vi "反控参数变更.vi"(11 "设置参数":T1(ring)=enum."CODMn") -> ()   [LabVIEW 2016, in "斯坦道CODMn新电路板.lvlib"]
panel:
  in  "错误输入（无错误）":errorcluster
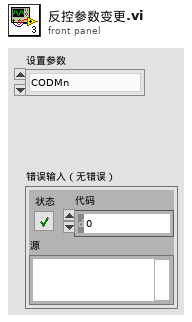
[diagram p1: front panel]
types:
  T1 = enum16{"", "CODMn", "PH", "氨氮", "总氮", "总磷", "CODCr", "电导率", "水温", "溶解氧", "浊度", "叶绿素", "藻密度", "ORP"}
  T2 = typedef "量程选择控件.ctl" = enum32{"L", "H", "AUTO"}
  T3 = typedef "操作日志字段定义.ctl" = cluster{"时间":timestamp, "参数":string, "日志信息":string, "流程参数":string}
  T4 = cluster{"水样测试量程模式":T2, "标样核查量程模式":T2, "零点核查量程模式":T2, "跨度核查量程模式":T2, "空白测试量程模式":T2, "平行样测试量程模式":T2, "加标回收量程模式":T2, "空白校准量程模式":T2, "标样校准量程模式":T2}
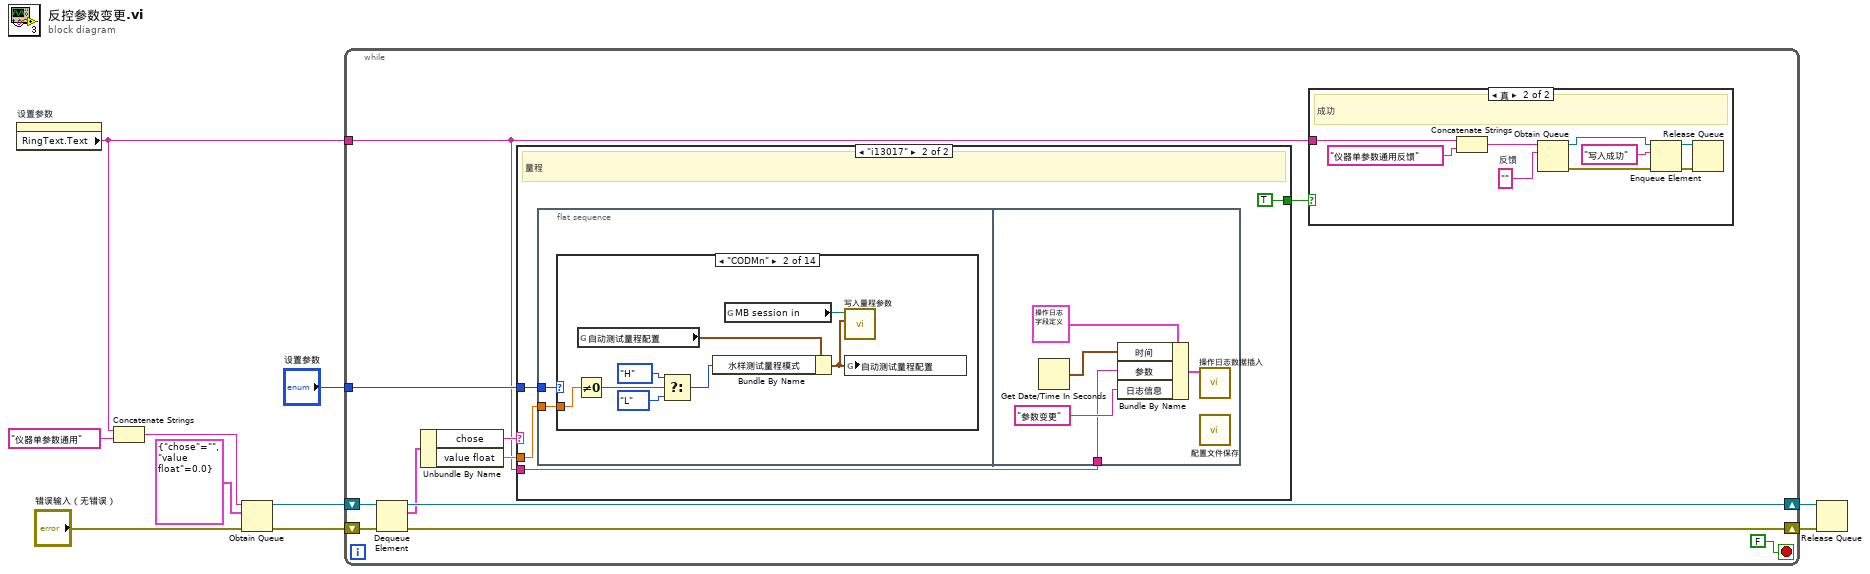
[diagram p0: block diagram]
diagram:
  n1 = property on="设置参数" class="Enum (严格)"() -> ("RingText.Text"=w2:string)  [unwired: 2 in, 2 out]
  n2 = Concatenate Strings(w2, "仪器单参数通用" ("名称（未命名）")) -> (w7:string)
  n3 = Obtain Queue(name (unnamed)=w7, element data type=cluster{"chose":string, "value float":dbl} {"chose"="", "value float"=0.0}, error in (no error)="错误输入（无错误）") -> (queue out=w6:refnum<queue>, error out=w5:errorcluster)  [unwired: 2 in, 1 out]
  n4 = while {
    shift-right: [w19] -> w4
    shift-left: w6 -> [w21]
    shift-right: [w18] -> w3
    shift-left: w5 -> [w20]
    tunnel: w2 -> [w11]
    tunnel: "设置参数" -> [w12]
    stop <- FALSE stop-if-true
    n5 = Dequeue Element(queue=w21, error in (no error)=w20) -> (queue out=w19:refnum<queue>, element=w16:cluster{"chose":string, "value float":dbl}, error out=w18:errorcluster)  [unwired: 1 in, 1 out]
    n6 = Unbundle By Name(w16) -> ("chose"=w15:string, "value float"=w13:dbl)
    n7 = case shown="\"i13017\"" w15 {
      tunnel: w13 -> [_ w32]
      tunnel: [_ TRUE] -> w14
      tunnel: w12 -> [_ w33]
      tunnel: w11 -> [_ w31]
      frame "假", Default {
      }
      frame "i13017" {
        # "量程"
        n8 = flat-sequence {
          tunnel: w33 -> [w36]
          tunnel: w32 -> [w35]
          tunnel: w31 -> [w46]
          frame #0 {
            n9 = case shown="\"CODMn\"" w36 {
              tunnel: w35 -> [_ w44 _ _ _ _ _ _ _ _ _ _ _ _]
              frame "", Default {
              }
              frame "CODMn" {
                n10 = Not Equal To 0?(x=w44) -> (x != 0?=w43:bool)
                n11 = global read "CODMn断电保存全局变量.vi" "自动测试量程配置"() -> (w40:T4)
                n12 = Select(t=量程选择控件."H" ("水样测试量程模式"), s=w43, f=量程选择控件."L" ("水样测试量程模式")) -> (s? t:f=w37:T2)
                n13 = Bundle By Name(cluster=w40, "水样测试量程模式"=w37) -> (w41:T4)
                n14 = global read "VARCODMn全局变量.vi" "MB session in"() -> (w39:refnum<class "MB_Master.lvclass">)
                n15 = call "写入量程参数.vi"("自动测试量程配置"=w41, "MB session in"=w39) -> ()  [unwired: 8 in, 2 out]
                n16 = global write "CODMn断电保存全局变量.vi" "自动测试量程配置"(w41) -> ()
              }
              frame "PH" {
              }
              frame "氨氮" {
              }
              frame "总氮" {
              }
              frame "总磷" {
              }
              frame "CODCr" {
              }
              frame "电导率" {
              }
              frame "水温" {
              }
              frame "溶解氧" {
              }
              frame "浊度" {
              }
              frame "叶绿素" {
              }
              frame "藻密度" {
              }
              frame "ORP" {
              }
            }
          }
          frame #1 {
            n17 = Get Date/Time In Seconds() -> (seconds since 1Jan1904=w48:timestamp)
            n18 = Bundle By Name(cluster=T3 {"时间"=timestamp(0 s since 1904-01-01), "参数"="", "日志信息"="", "流程参数"=""} ("data in"), "时间"=w48, "参数"=w46, "日志信息"="参数变更") -> (w45:T3)
            n19 = call "操作日志数据插入.vi"("data"=w45) -> ()  [unwired: 9 in, 1 out]
            n20 = call "配置文件保存.vi"() -> ()  [unwired: 12 in]
          }
        }
      }
    }
    n21 = case shown="真" w14 {
      tunnel: w11 -> [_ w29]
      frame False {
      }
      frame True {
        w24 = ""  # 反馈
        # "成功"
        n22 = Concatenate Strings(w29, "仪器单参数通用反馈" ("名称（未命名）")) -> (w23:string)
        n23 = Obtain Queue(name (unnamed)=w23, element data type=w24) -> (queue out=w25:refnum<queue>, error out=w26:errorcluster)  [unwired: 3 in, 1 out]
        n24 = Enqueue Element(queue=w25, element="写入成功" ("元素"), error in (no error)=w26) -> (queue out=w28:refnum<queue>, error out=w27:errorcluster)  [unwired: 1 in, 1 out]
        n25 = Release Queue(queue=w28, error in (no error)=w27) -> ()  [unwired: 1 in, 3 out]
      }
    }
  }
  n26 = Release Queue(queue=w4, error in (no error)=w3) -> ()  [unwired: 1 in, 3 out]
